vi "PH_OceanOpticsSpectrometer.constructor.vi"(0 "name":string, 2 "data in":string, 5 "error in(no error)":errorcluster) -> (14 "i ref out":refnum<vi>, 16 "data out":string, 19 "error out":errorcluster)   [LabVIEW 2014, in "PH_OceanOpticsSpectrometer.lvlib"]
doc: "This class is forseen to operate an Ocean Optics spectrometer (Typ HR2000+ or HR4000). \n\nThis class is part of the PHELIX device layer.\n\nauthor: Stefan Götte, GSI\n\nLicense Agreement for this software:\n\nCopyright (C)\nGesellschaft für Schwerionenforschung, GSI\nPlanckstr. 1\n64291 Darmstadt\nGermany\n\nContact: D.Beck@gsi.de \n\nThis program is free software; you can redistribute it and/or modify it under the terms of the \nGNU General Public License as published by the Free Software Foundation; either version 2 of \nthe license, or (at your option) any later version.\n\nThis program is distributed in the hope that it will be useful, but WITHOUT ANY WARRANTY; \nwithout even the implied warranty of MERCHANTABILITY or FITNESS FOR A PARTICULAR PURPOSE. See the GNU General License for more details (http://www.gnu.org).\n\nGesellschaft für Schwerionenforschung, GSI\nPlanckstr. 1, 64291 Darmstadt, Germany\nFor all questions and ideas contact: M.Richter@gsi.de, H.Brand@gsi.de or D.Beck@gsi.de.\nLast update: 16-JUN-2004"
uses:
  PH_OceanOpticsSpectrometer.lvlib
  CS_Core/BaseProcess/BaseProcess.lvlib
  PH_Basics/PH_PSDBWriter/PH_PSDBWriter.lvlib
  PH_Basics/PH_Class/PH_Class.lvlib
  PH_Basics/PH_StatusHandler/PH_StatusHandler.lvlib
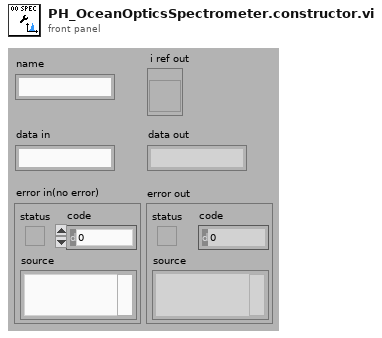
[diagram p1: front panel]
types:
  T1 = enum16{"SetAttribute", "GetAttribute", "CreateAttribute", "DestroyAttribute", "DestroyAllAtributes"}
  T2 = typedef "PH_OceanOpticsSpectrometer.lvlib/PH_OceanOpticsSpectrometer.i attribute.ctl" = cluster{"GUI Refs":cluster{"Delete":refnum<vi>, "Spectrum":refnum<vi>, "Display Width":refnum<vi>, "Display Center":refnum<vi>, "Save":refnum<vi>, "Integration time":refnum<vi>, "center wavelength":refnum<vi>, "width":refnum<vi>, "Wanted Trigger Mode":refnum<vi>, "Current Trigger Mode":refnum<vi>, "Trigger Info":refnum<vi>, "Model":refnum<vi>, "Driver":refnum<vi>, "Firmware":refnum<vi>}, "Display":cluster{"Width":dbl, "Center":dbl}, "VISA resource name":refnum<visa-resource-name>, "Integration time [ms]":cluster{"Current Value":u16, "Wanted Value":u16}, "Trigger":cluster{"Current value":T3, "Wanted value":T3}, "Default VISA Timeout":u32, "Last Data":cluster{"Wavelength Bins":dbl[], "Spectrum by Pixels":dbl[]}}
  T3 = typedef "PH_OceanOpticsSpectrometer.lvlib/PH_OceanOpticsSpectrometer.Trigger.ctl" = enum32{"External", "Normal"}
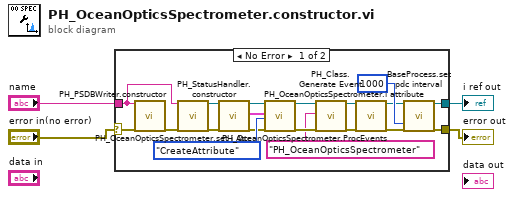
[diagram p0: block diagram]
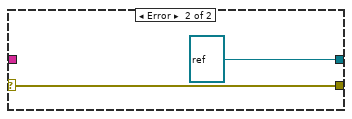
[diagram p2: hidden frame]
diagram:
  n1 = case shown="No Error" "error in(no error)" {
    selector: "error in(no error)" -> [w23 w25]
    tunnel: "name" -> [w5 _]
    tunnel: [w21 refnum<vi> refnum ("i ref out")] -> w3
    tunnel: [w20 w25] -> w2
    frame No Error {
      n2 = call "PH_PSDBWriter.constructor.vi"("name"=w5, "error in"=w23) -> ("error out"=w11:errorcluster)  [unwired: 15 in, 2 out]
      n3 = call "PH_StatusHandler.constructor.vi"("name"=w5, "error in(no error)"=w11) -> ("i ref out"=w6:refnum<vi>, "error out"=w7:errorcluster)  [unwired: 15 in, 1 out]
      n4 = call "PH_OceanOpticsSpectrometer.set i Attr.vi"("i ref in"=w6, "error in (no error)"=w7) -> ("i ref out"=w9:refnum<vi>, "i Attributes"=w10:T2, "error out"=w8:errorcluster)  [unwired: 15 in]
      n5 = call "PH_OceanOpticsSpectrometer.i attribute.vi"("VI Refnum"=w9, "CLASS.i attribute"=w10, "Action"=T1."CreateAttribute", "error in (no error)"=w8) -> ("VI Refnum out"=w14:refnum<vi>, "error out"=w13:errorcluster)  [unwired: 13 in, 1 out]
      n6 = call "PH_Class.Generate Event.vi"("i ref in"=w14, "Class"="PH_OceanOpticsSpectrometer", "error in (no error)"=w13) -> ("i ref out"=w17:refnum<vi>, "error out"=w16:errorcluster)  [unwired: 15 in]
      n7 = call "PH_OceanOpticsSpectrometer.ProcEvents.vi"("i ref in"=w17, "error in"=w16) -> ("i ref out"=w19:refnum<vi>, "error out"=w18:errorcluster)  [unwired: 16 in]
      n8 = call "BaseProcess.set pdc interval.vi"("i ref in"=w19, "PeriodicInterval [ms]"=1000, "error in (no error)"=w18) -> ("i ref out"=w21:refnum<vi>, "error out"=w20:errorcluster)  [unwired: 14 in, 1 out]
    }
    frame Error {
    }
  }
  "i ref out" <- w3
  "error out" <- w2
